vi "close Serial port.vi"(8 "error in (no error)":errorcluster caption="错误输入（无错误）", 11 "BD Protocol 4.0 输入":refnum<class "BD Protocol 4.0.lvclass">) -> (0 "error out":errorcluster caption="错误输出", 3 "BD Protocol 4.0 输出":refnum<class "BD Protocol 4.0.lvclass">)   [LabVIEW 2016, in "BD Protocol 4.0.lvlib" / "BD Protocol 4.0.lvclass"]
uses:
  BD Protocol 4.0.lvclass
  BD Protocol 4.0.lvclass/BD Protocol 4.0.ctl
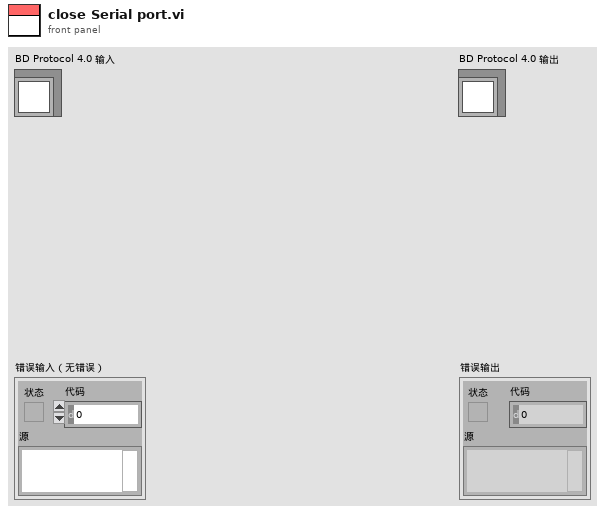
[diagram p1: front panel]
types:
  T1 = enum8{"Enabled", "Disabled", "Disabled and Grayed Out"}
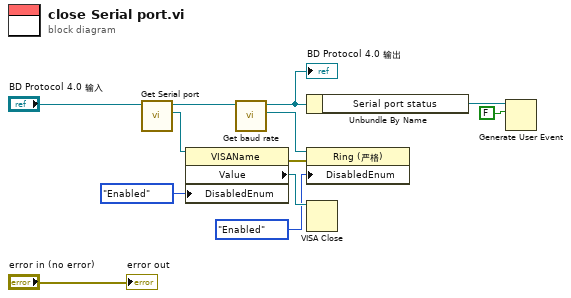
[diagram p0: block diagram]
diagram:
  n1 = call "Get Serial port.vi"("BD Protocol 4.0 in"="BD Protocol 4.0 输入") -> ("Serial port"=w10:refnum<vi>, "BD Protocol 4.0 out"=w9:refnum<class "BD Protocol 4.0.lvclass">)  [unwired: 9 in]
  n2 = property class="VISAName"(reference=w10, "DisabledEnum"=T1."Enabled" ("禁用")) -> (error out=w4:errorcluster, "Value"=w8:refnum<visa-resource-name>)  [unwired: 1 in, 1 out]
  n3 = call "Get baud rate.vi"("BD Protocol 4.0 in"=w9) -> ("baud rate"=w6:refnum<vi>, "BD Protocol 4.0 out"=w3:refnum<class "BD Protocol 4.0.lvclass">)  [unwired: 9 in]
  "BD Protocol 4.0 输出" <- w3
  n4 = Unbundle By Name(w3) -> ("Serial port status"=w2:refnum<user-event>)
  n5 = property class="Ring (严格)"(reference=w6, error in=w4, "DisabledEnum"=T1."Enabled" ("禁用")) -> ()  [unwired: 2 out]
  n6 = VISA Close(VISA resource name=w8) -> ()  [unwired: 1 in, 1 out]
  n7 = Generate User Event(user event=w2, event data cluster=FALSE ("事件数据")) -> ()  [unwired: 2 in, 2 out]
  "error out" <- "error in (no error)"
